vi "数据读取.vi"(8 "error out":errorcluster, 9 "输入字符串":string, 11 "VISA resource name out":refnum<visa-resource-name>) -> (0 "error out 2":errorcluster caption="error out", 1 "输出字符串":string, 2 "数组 3":sgl[](array[numeric]), 3 "VISA resource name out 2":refnum<visa-resource-name>, 4 "布尔":bool=TRUE)   [LabVIEW 2020]
panel:
  out "所有小写字母字符串":string
  out "数组 2":i32[](array[numeric])
  out "数组":string[](array[string])
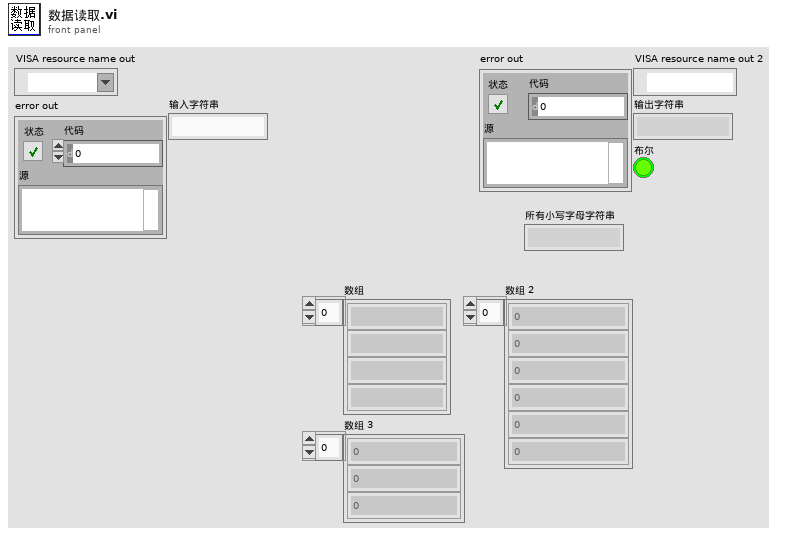
[diagram p1: front panel]
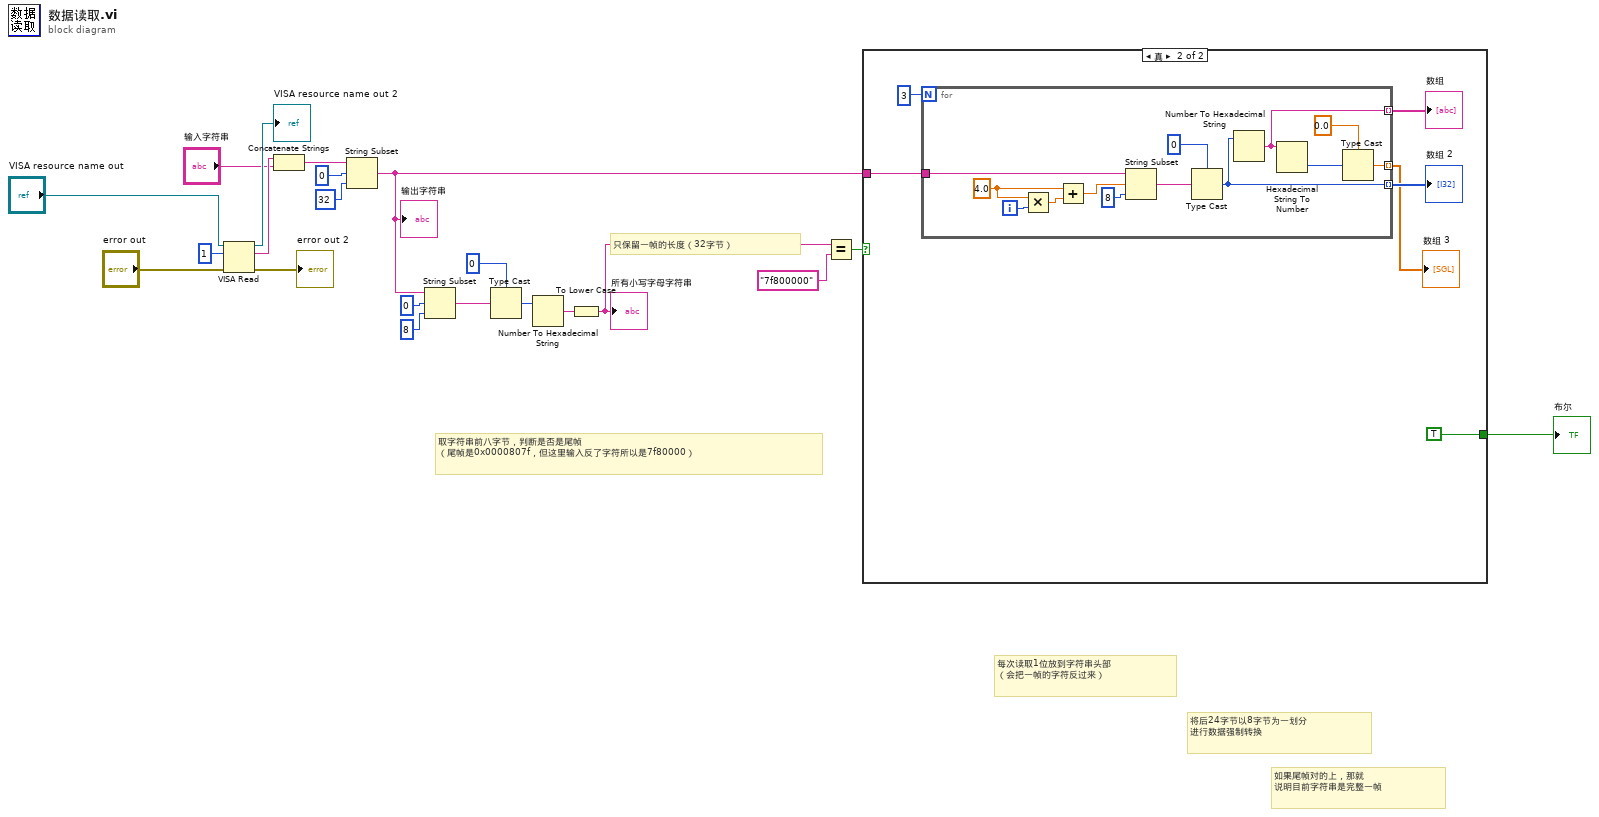
[diagram p0: block diagram]
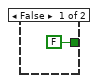
[diagram p2: hidden frame]
diagram:
  # "将后24字节以8字节为一划分\n进行数据强制转换"
  # "如果尾帧对的上，那就\n说明目前字符串是完整一帧"
  # "只保留一帧的长度（32字节）"
  # "取字符串前八字节，判断是否是尾帧\n（尾帧是0x0000807f，但这里输入反了字符所以是7f80000）"
  # "每次读取1位放到字符串头部\n（会把一帧的字符反过来）"
  n1 = VISA Read(VISA resource name="VISA resource name out", byte count=u32 1 ("字节总数"), error in (no error)="error out") -> (VISA resource name out=→"VISA resource name out 2":refnum<visa-resource-name>, read buffer=w18:string, error out=→"error out 2":errorcluster)  [unwired: 1 out]
  n2 = Concatenate Strings(w18, "输入字符串") -> (w14:string)
  n3 = String Subset(string=w14, offset (0)=0 ("偏移量(0)"), length (rest)=32 ("长度（剩余）")) -> (substring=w21:string)
  "输出字符串" <- w21
  n4 = String Subset(string=w21, offset (0)=0 ("偏移量(0)"), length (rest)=8 ("长度（剩余）")) -> (substring=w15:string)
  n5 = Type Cast(type=0 ("长度（剩余）"), x=w15) -> (*(type *) &x=w16:i32)
  n6 = Number To Hexadecimal String(2:w16) -> (0:w17:string)  [unwired: 1 in]
  n7 = To Lower Case(string=w17) -> (all lower case string=w19:string)
  "所有小写字母字符串" <- w19
  n8 = Equal?(x=w19, y="7f800000") -> (x = y?=w20:bool)
  n9 = case shown="真" w20 {
    tunnel: w21 -> [_ w25]
    tunnel: [FALSE TRUE] -> w1
    frame False {
    }
    frame True {
      n10 = for {
        N: 3 -> [_]
        tunnel: [w39] -> w28 mode=indexing
        tunnel: [w36] -> w27 mode=indexing
        tunnel: w25 -> [w37]
        tunnel: [w33] -> w24 mode=indexing
        i -> [w31]
        w29 = 4.0 ("x")
        n11 = Multiply(x=w29, y=w31) -> (x*y=w30:dbl)
        n12 = Add(x=w29, y=w30) -> (x+y=w32:dbl)
        n13 = String Subset(string=w37, offset (0)=w32, length (rest)=8 ("长度（剩余）")) -> (substring=w38:string)
        n14 = Type Cast(type=0 ("长度（剩余）"), x=w38) -> (*(type *) &x=w39:i32)
        n15 = Number To Hexadecimal String(2:w39) -> (0:w36:string)  [unwired: 1 in]
        n16 = Hexadecimal String To Number(string=w36) -> (number=w34:u32)  [unwired: 2 in, 1 out]
        n17 = Type Cast(type=sgl 0.0, x=w34) -> (*(type *) &x=w33:sgl)
      }
      "数组 2" <- w28
      "数组" <- w27
      "数组 3" <- w24
    }
  }
  "布尔" <- w1
